vi "Initialize.vi"(7 "thread ID":i32, 8 "error in (no error)":errorcluster, 9 "component name":string, 10 "Plugin Configuration":refnum<class "Plugin Configuration.lvclass">, 11 "Type Converter in":refnum<class "Default Buffer Converter.lvclass">) -> (0 "error out":errorcluster, 3 "Type Converter out":refnum<class "Default Buffer Converter.lvclass">)   [LabVIEW 2019, in "DSF Core.lvlib" / "Default Buffer Converter.lvclass"]
uses:
  Default Buffer Converter.lvclass
  Classes/Configuration/Core/Plugin/Plugin Configuration.lvclass
  Classes/Configuration/Core/Plugin/Plugin Configuration.lvclass/Plugin Configuration.ctl
  Classes/Configuration/Core/Thread/Thread Configuration.lvclass/Thread Configuration.ctl
  Default Buffer Converter.lvclass/Default Buffer Converter.ctl
  Conversion.ctl
  Conversion Block.ctl
  Typedefs/DSF Data Type.ctl
  Classes/Configuration/Core/Group/Group Configuration.lvclass/Group Configuration.ctl
  Configurations/Default Buffer Converter Transfer Configuration.lvclass
  Classes/Configuration/Core/Core Configuration.lvclass/Core Configuration.ctl
  Classes/Configuration/Core/Transfer/Transfer Configuration.lvclass
  C:/Dev/GitHub/niveristand-data-sharing-framework-custom-device/Core/Classes/Configuration/Core/Core Configuration.lvclass
  Classes/Configuration/Core/Group/Group Configuration.lvclass
  DSF Core.lvlib
  Classes/Configuration/Core/Thread/Thread Configuration.lvclass
  Classes/Configuration/Core/Core Configuration.lvclass
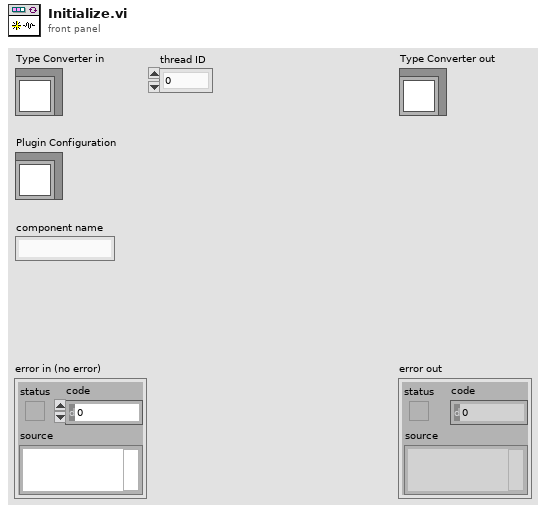
[diagram p1: front panel]
types:
  T1 = typedef "DSF Core.lvlib/Default Buffer Converter.lvclass/Conversion.ctl" = cluster{"conversion blocks":T2[]}
  T2 = typedef "DSF Core.lvlib/Default Buffer Converter.lvclass/Conversion Block.ctl" = cluster{"engine offset":u64, "engine data type":T3, "string offset":u64, "string data type":T3, "engine byte order":enum16{"big-endian, network order", "native, host order", "little-endian"}, "string byte order":enum16{"big-endian, network order", "native, host order", "little-endian"}, "count":u64}
  T3 = typedef "DSF Core.lvlib/DSF Data Type.ctl" = enum8{"Bool", "SGL", "DBL", "I8", "I16", "I32", "I64", "U8", "U16", "U32", "U64"}
  T4 = typedef "DSF Core.lvlib/DSF Settings Info.ctl" = cluster{"component":string, "values":cluster{"key":string, "value":string}[]}
  T5 = typedef "DSF Core.lvlib/Default Buffer Converter Transfer Configuration.lvclass/Transfer Configuration.ctl" = cluster{"byte order":T6}
  T6 = typedef "DSF Core.lvlib/DSF Byte Order.ctl" = enum8{"big-endian", "little-endian"}
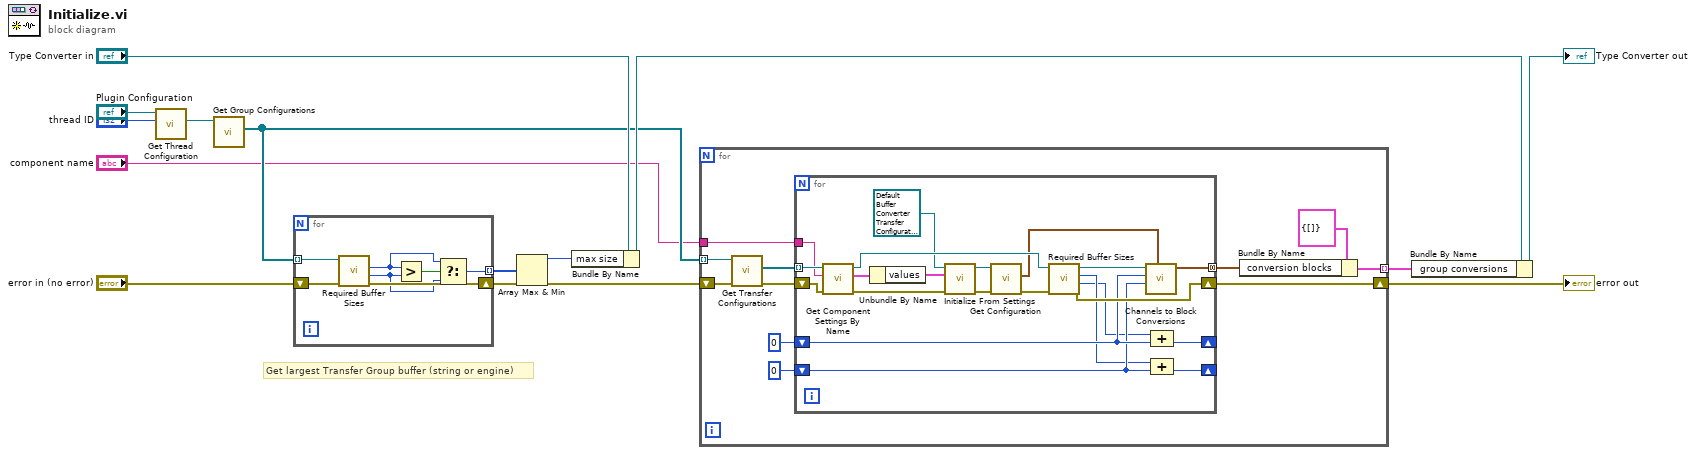
[diagram p0: block diagram]
diagram:
  # "Get largest Transfer Group buffer (string or engine)"
  n1 = call "Get Thread Configuration.vi"("index"="thread ID", "Plugin Configuration in"="Plugin Configuration") -> ("Thread Configuration"=w4:refnum<class "Thread Configuration.lvclass">)  [unwired: 7 in, 2 out]
  n2 = call "Get Group Configurations.vi"("Thread Configuration in"=w4) -> ("Group Configurations"=w7:refnum<class "Group Configuration.lvclass">[])  [unwired: 8 in, 2 out]
  n3 = for {
    tunnel: w7 -> [w19] mode=indexing
    tunnel: [w20] -> w14 mode=indexing
    shift-right: [w16] -> w2
    shift-left: "error in (no error)" -> [w18]
    n4 = call-dynamic "Required Buffer Sizes.vi"("error in (no error)"=w18, "Group Configuration in"=w19) -> ("error out"=w16:errorcluster, "string size"=w15:u64, "engine size"=w17:u64)  [unwired: 6 in, 1 out]
    n5 = Greater?(x=w17, y=w15) -> (0:w21:bool)
    n6 = Select(t=w17, s=w21, f=w15) -> (s? t:f=w20:u64)
  }
  n7 = Array Max & Min(array=w14) -> (max value=w8:u64)  [unwired: 3 out]
  n8 = Bundle By Name(cluster="Type Converter in", "max size"=w8) -> (w9:refnum<class "Default Buffer Converter.lvclass">)
  n9 = for {
    tunnel: w7 -> [w27] mode=indexing
    tunnel: [w30] -> w12 mode=indexing
    tunnel: "component name" -> [w25]
    shift-right: [w22] -> w1
    shift-left: w2 -> [w24]
    n10 = call "Get Transfer Configurations.vi"("error in (no error)"=w24, "Group Configuration in"=w27) -> ("error out"=w23:errorcluster, "Transfer Configurations"=w26:refnum<class "Transfer Configuration.lvclass">[])  [unwired: 7 in, 1 out]
    n11 = for {
      tunnel: w26 -> [w44] mode=indexing
      tunnel: [w52] -> w31 mode=concatenating
      shift-right: [w51] -> _
      shift-left: u64 0 ("engine buffer size") -> [w49]
      shift-right: [w50] -> _
      shift-left: u64 0 ("engine buffer size") -> [w48]
      tunnel: w25 -> [w43]
      shift-right: [w53] -> w22
      shift-left: w23 -> [w35]
      n12 = call "Get Component Settings By Name.vi"("error in (no error)"=w35, "component name"=w43, "Runtime Configuration in"=w44) -> ("error out"=w38:errorcluster, "component settings"=w42:T4, "Runtime Configuration out"=w37:refnum<class "Transfer Configuration.lvclass">)  [unwired: 6 in]
      n13 = Unbundle By Name(w42) -> ("values"=w40:cluster{"key":string, "value":string}[])
      n14 = call-dynamic "Initialize From Settings.vi"("error in (no error)"=w38, "settings"=w40, "DSF Buffer Converter Transfer Configuration in"=refnum<class "Default Buffer Converter Transfer Configuration.lvclass"> refnum) -> ("error out"=w39:errorcluster, "DSF Buffer Converter Transfer Configuration out"=w41:refnum<class "Default Buffer Converter Transfer Configuration.lvclass">)  [unwired: 7 in]
      n15 = call "Get Configuration.vi"("error in (no error)"=w39, "DSF Buffer Converter Transfer Configuration in"=w41) -> ("error out"=w36:errorcluster, "configuration"=w33:T5)  [unwired: 7 in, 1 out]
      n16 = call-dynamic "Required Buffer Sizes.vi"("error in (no error)"=w36, "Transfer Configuration in"=w37) -> ("error out"=w53:errorcluster, "string size"=w45:u64, "engine size"=w46:u64, "Transfer Configuration out"=w47:refnum<class "Transfer Configuration.lvclass">)  [unwired: 6 in]
      n17 = call "Channels to Block Conversions.vi"("transfer configuration"=w33, "initial engine buffer offset"=w48, "initial string buffer offset"=w49, "Transfer Configuration"=w47) -> ("Transfer conversion descriptors"=w52:T2[])  [unwired: 7 in]
      n18 = Compound Arithmetic op=ADD(w45, w49) -> (w51:u64)
      n19 = Compound Arithmetic op=ADD(w46, w48) -> (w50:u64)
    }
    n20 = Bundle By Name(cluster=T1 {"conversion blocks"=[]} ("conversion"), "conversion blocks"=w31) -> (w30:T1)
  }
  "error out" <- w1
  n21 = Bundle By Name(cluster=w9, "group conversions"=w12) -> (→"Type Converter out":refnum<class "Default Buffer Converter.lvclass">)
